vi "Main.vi"() -> ()   [LabVIEW 2012]
uses:
  Consumer Message.ctl
panel:
  out "Consumer Shutdown?":bool
  out "State to Execute":string
  out "High Priority?":bool
  out "Backlog":u8(slide) scale=0.0..100.0
  out "Processed Value":i32
  in  "High Priority Message":bool
  in  "Normal Priority Message":bool
  in  "Stop":bool
  # "Number of enqueued messages waiting to be processed"
  # "Current data being processed in consumer loop"
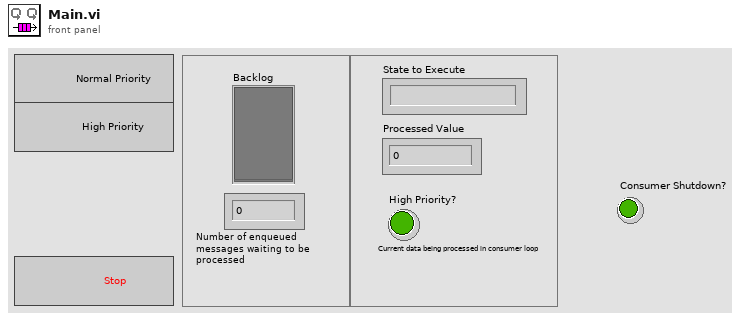
[diagram p1: front panel]
types:
  T1 = typedef "Consumer Message.ctl" = cluster{"Consumer State":string, "Boolean Data":bool, "Numeric Data":i32, "Error":errorcluster}
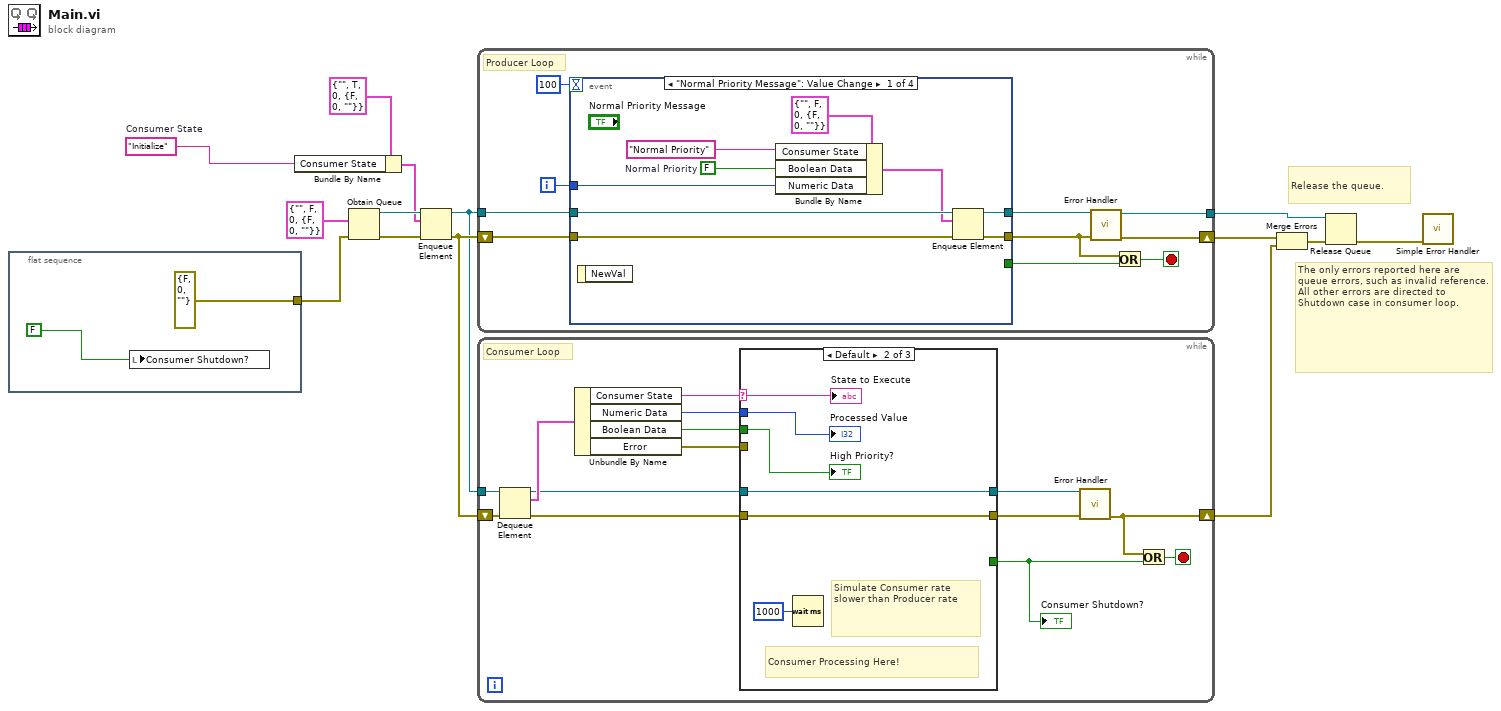
[diagram p0: block diagram]
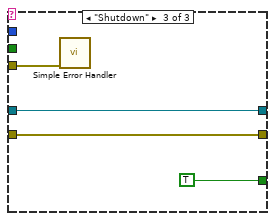
[diagram p3: hidden frame]
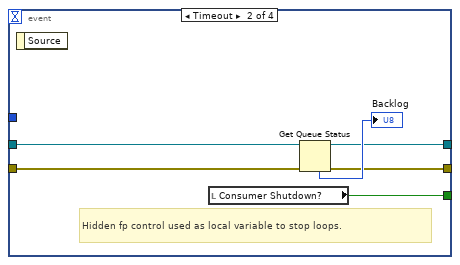
[diagram p4: hidden frame]
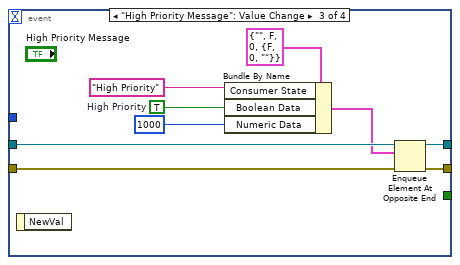
[diagram p5: hidden frame]
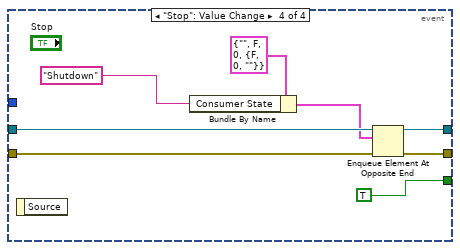
[diagram p6: hidden frame]
diagram:
  w6 = "Initialize"  # Consumer State
  # "Release the queue."
  # "The only errors reported here are queue errors, such as invalid reference.  All other errors are directed to Shutdown case in consumer loop."
  n1 = flat-sequence {
    tunnel: [errorcluster {"status"=FALSE, "code"=0, "source"=""} ("error in (no error)")] -> w9
    frame #0 {
      n2 = local write "Consumer Shutdown?"(FALSE ("Stop Loops (local)")) -> ()
    }
  }
  n3 = Bundle By Name(cluster=T1 {"Consumer State"="", "Boolean Data"=TRUE, "Numeric Data"=0, "Error"={"status"=FALSE, "code"=0, "source"=""}} ("Consumer Message"), "Consumer State"=w6) -> (w7:T1)
  n4 = Obtain Queue(element data type=T1 {"Consumer State"="", "Boolean Data"=FALSE, "Numeric Data"=0, "Error"={"status"=FALSE, "code"=0, "source"=""}}, error in (no error)=w9) -> (queue out=w11:refnum<queue>, error out=w14:errorcluster)  [unwired: 3 in, 1 out]
  n5 = Enqueue Element(queue=w11, element=w7, error in (no error)=w14) -> (queue out=w10:refnum<queue>, error out=w12:errorcluster)  [unwired: 1 in, 1 out]
  n6 = while {
    tunnel: w10 -> [w26]
    shift-right: [w18] -> w5
    shift-left: w12 -> [w25]
    tunnel: [w17] -> w1
    i -> [w24]
    stop <- w20 stop-if-true
    # "Producer Loop"
    n7 = event shown="[0] \"Normal Priority Message\": Value Change" {
      selector: _ -> [_ _ _ _]
      dyn-events: _ -> [_ _ _ _]
      timeout: 100 -> [_ _ _ _]
      tunnel: w26 -> [w35 w39 w49 w58]
      tunnel: w25 -> [w33 w38 w48 w56]
      tunnel: [w34 w37 w50 w55] -> w19
      tunnel: [_ w41 _ TRUE] -> w21
      tunnel: w24 -> [w32 _ _ _]
      tunnel: [w28 w36 w44 w54] -> w23
      event "Normal Priority Message": Value Change {
        w29 = FALSE  # Normal Priority
        n8 = event-data() -> ()  [unwired: 1 in, 1 out]
        n9 = Bundle By Name(cluster=T1 {"Consumer State"="", "Boolean Data"=FALSE, "Numeric Data"=0, "Error"={"status"=FALSE, "code"=0, "source"=""}}, "Consumer State"="Normal Priority" ("String Data"), "Boolean Data"=w29, "Numeric Data"=w32) -> (w31:T1)
        n10 = Enqueue Element(queue=w35, element=w31, error in (no error)=w33) -> (queue out=w28:refnum<queue>, error out=w34:errorcluster)  [unwired: 1 in, 1 out]
      }
      event Timeout {
        # "Hidden fp control used as local variable to stop loops."
        n11 = event-data() -> ()  [unwired: 1 in, 1 out]
        n12 = local read "Consumer Shutdown?"() -> (w41:bool)
        n13 = Get Queue Status(queue=w39, error in (no error)=w38) -> (queue out=w36:refnum<queue>, error out=w37:errorcluster, # elements in queue=→"Backlog":i32)  [unwired: 1 in, 5 out]
      }
      event "High Priority Message": Value Change {
        w43 = TRUE  # High Priority
        n14 = event-data() -> ()  [unwired: 1 in, 1 out]
        n15 = Bundle By Name(cluster=T1 {"Consumer State"="", "Boolean Data"=FALSE, "Numeric Data"=0, "Error"={"status"=FALSE, "code"=0, "source"=""}}, "Consumer State"="High Priority" ("String Data"), "Boolean Data"=w43, "Numeric Data"=1000) -> (w46:T1)
        n16 = Enqueue Element At Opposite End(queue=w49, element=w46, error in (no error)=w48) -> (queue out=w44:refnum<queue>, error out=w50:errorcluster)  [unwired: 1 in, 1 out]
      }
      event "Stop": Value Change {
        n17 = event-data() -> ()  [unwired: 1 in, 1 out]
        n18 = Bundle By Name(cluster=T1 {"Consumer State"="", "Boolean Data"=FALSE, "Numeric Data"=0, "Error"={"status"=FALSE, "code"=0, "source"=""}}, "Consumer State"="Shutdown") -> (w51:T1)
        n19 = Enqueue Element At Opposite End(queue=w58, element=w51, error in (no error)=w56) -> (queue out=w54:refnum<queue>, error out=w55:errorcluster)  [unwired: 1 in, 1 out]
      }
    }
    n20 = call "Error Handler.vi"("error in"=w19, "queue in"=w23) -> ("error out"=w18:errorcluster, "queue out"=w17:refnum<queue>)  [unwired: 8 in]
    n21 = Or(x=w19, y=w21) -> (x .or. y?=w20:bool)
  }
  n22 = while {
    tunnel: w10 -> [w72]
    shift-right: [w61] -> w4
    shift-left: w12 -> [w71]
    stop <- w62 stop-if-true
    # "Consumer Loop"
    n23 = Dequeue Element(queue=w72, error in (no error)=w71) -> (queue out=w60:refnum<queue>, element=w70:T1, error out=w59:errorcluster)  [unwired: 1 in, 1 out]
    n24 = Unbundle By Name(w70) -> ("Consumer State"=w69:string, "Numeric Data"=w68:i32, "Boolean Data"=w67:bool, "Error"=w64:errorcluster)
    n25 = case shown="Default" w69 {
      selector: w69 -> [_ w77 _]
      tunnel: [_ _ TRUE] -> w63
      tunnel: w59 -> [w73 w75 w81]
      tunnel: [w73 w75 w81] -> w66
      tunnel: w68 -> [_ w80 _]
      tunnel: w67 -> [_ w79 _]
      tunnel: w60 -> [w74 w78 w82]
      tunnel: [w74 w78 w82] -> w65
      tunnel: w64 -> [_ _ w83]
      frame "Initialize" {
      }
      frame Default {
        # "Simulate Consumer rate slower than Producer rate"
        # "Consumer Processing Here!"
        n26 = Wait (ms)(milliseconds to wait=u32 1000) -> ()  [unwired: 1 out]
        "Processed Value" <- w80
        "High Priority?" <- w79
        "State to Execute" <- w77
      }
      frame "Shutdown" {
        n27 = call <vilib>:"Simple Error Handler.vi"("error in (no error)"=w83) -> ()  [unwired: 4 in, 5 out]
      }
    }
    "Consumer Shutdown?" <- w63
    n28 = call "Error Handler.vi"("error in"=w66, "queue in"=w65) -> ("error out"=w61:errorcluster)  [unwired: 8 in, 1 out]
    n29 = Or(x=w61, y=w63) -> (x .or. y?=w62:bool)
  }
  n30 = Merge Errors(w5, w4) -> (w3:errorcluster)
  n31 = Release Queue(queue=w1, error in (no error)=w3) -> (error out=w2:errorcluster)  [unwired: 1 in, 2 out]
  n32 = call <vilib>:"Simple Error Handler.vi"("error in (no error)"=w2) -> ()  [unwired: 4 in, 5 out]
